vi "XGB 통신.vi"(8 "error in (no error)":errorcluster, 10 "String":string, 11 "VISA Refnum in":refnum<visa-resource-name>) -> (0 "error out":errorcluster, 1 "Bytes at Port":u32, 2 "read buffer":string, 3 "VISA Refnum out":refnum<visa-resource-name>)   [LabVIEW 2014]
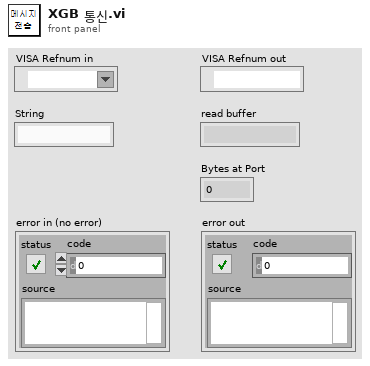
[diagram p1: front panel]
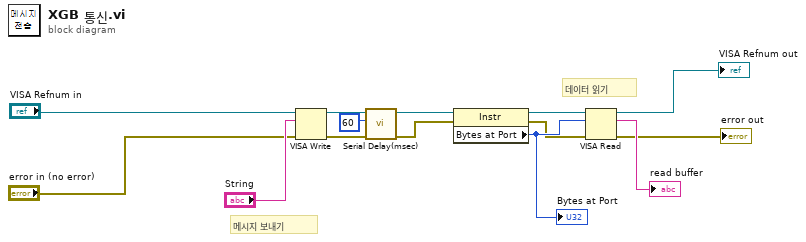
[diagram p0: block diagram]
diagram:
  # "데이터 읽기"
  # "메시지 보내기"
  n1 = VISA Write(VISA resource name="VISA Refnum in", write buffer="String", error in (no error)="error in (no error)") -> (VISA resource name out=w5:refnum<visa-resource-name>, error out=w2:errorcluster)  [unwired: 1 out]
  n2 = call "Serial Delay(msec).vi"("에러 입력(에러 없음)"=w2, "milliseconds to wait"=u32 60, "VISA 참조 번호 입력"=w5) -> ("에러 출력"=w3:errorcluster, "VISA 참조 번호 출력"=w4:refnum<visa-resource-name>)  [unwired: 7 in]
  n3 = property class="Instr"(reference=w4, error in=w3) -> (reference out=w7:refnum<visa-resource-name>, error out=w8:errorcluster, "Bytes at Port"=w13:u32)
  "Bytes at Port" <- w13
  n4 = VISA Read(VISA resource name=w7, byte count=w13, error in (no error)=w8) -> (VISA resource name out=→"VISA Refnum out":refnum<visa-resource-name>, read buffer=→"read buffer":string, error out=→"error out":errorcluster)  [unwired: 1 out]
